vi "VisualCheckSubPanel.vi"(6 "GuiRef":T1={"StringOut"=refnum, "AbortOnFail"=refnum, "SN"=refnum, "SN_Length"=refnum, "TestResult"=refnum, "CycleTime"=refnum, "ErrorCode"=refnum, "UUTStatus"=refnum, "DataBaseEnable?"=refnum, "DUTModel"=refnum, "FixtureID"=refnum, "OperatorID"=refnum, "SNReady"=refnum, "StopSlot"=refnum, "NextStep"=refnum, "PassYeild"=refnum, "Failed"=refnum, "Passed"=refnum, "Tested"=refnum, "TestItemsCtl"={"StepName"="", "TestEnable"=FALSE, "LoopCount"=0, "StopOnFail"=FALSE, "Index"=0, "TestName"="", "通道"="", "参数"="", "TimeStart"=0}, "ProcessBar"=refnum, "Slot"=enum."Slot1", "Row"=3, "States"=refnum, "TestMode"=refnum, "循环次数-DUT"=refnum, "波形图"=refnum, "产品型号"=refnum, "子面板"=refnum, "测试失败项目"=refnum, "测试结果"=refnum, "DUT"=refnum, "Starttime"=refnum, "SlotReady"=refnum, "版本信息"=refnum, "WIFI_1"=refnum, "WIFI_2"=refnum, "直通率"=refnum, "卡1开卡结果"=refnum, "卡2开卡结果"=refnum}, 8 "error in (no error)":errorcluster, 10 "测试项":string) -> (0 "error out":errorcluster, 2 "StringOut":string, 3 "Result":bool)   [LabVIEW 2013]
uses:
  SystemCode/SysControl/Reference.ctl
  SystemCode/SysControl/TestItemsCTL.ctl
  SystemCode/SysControl/Slot.ctl
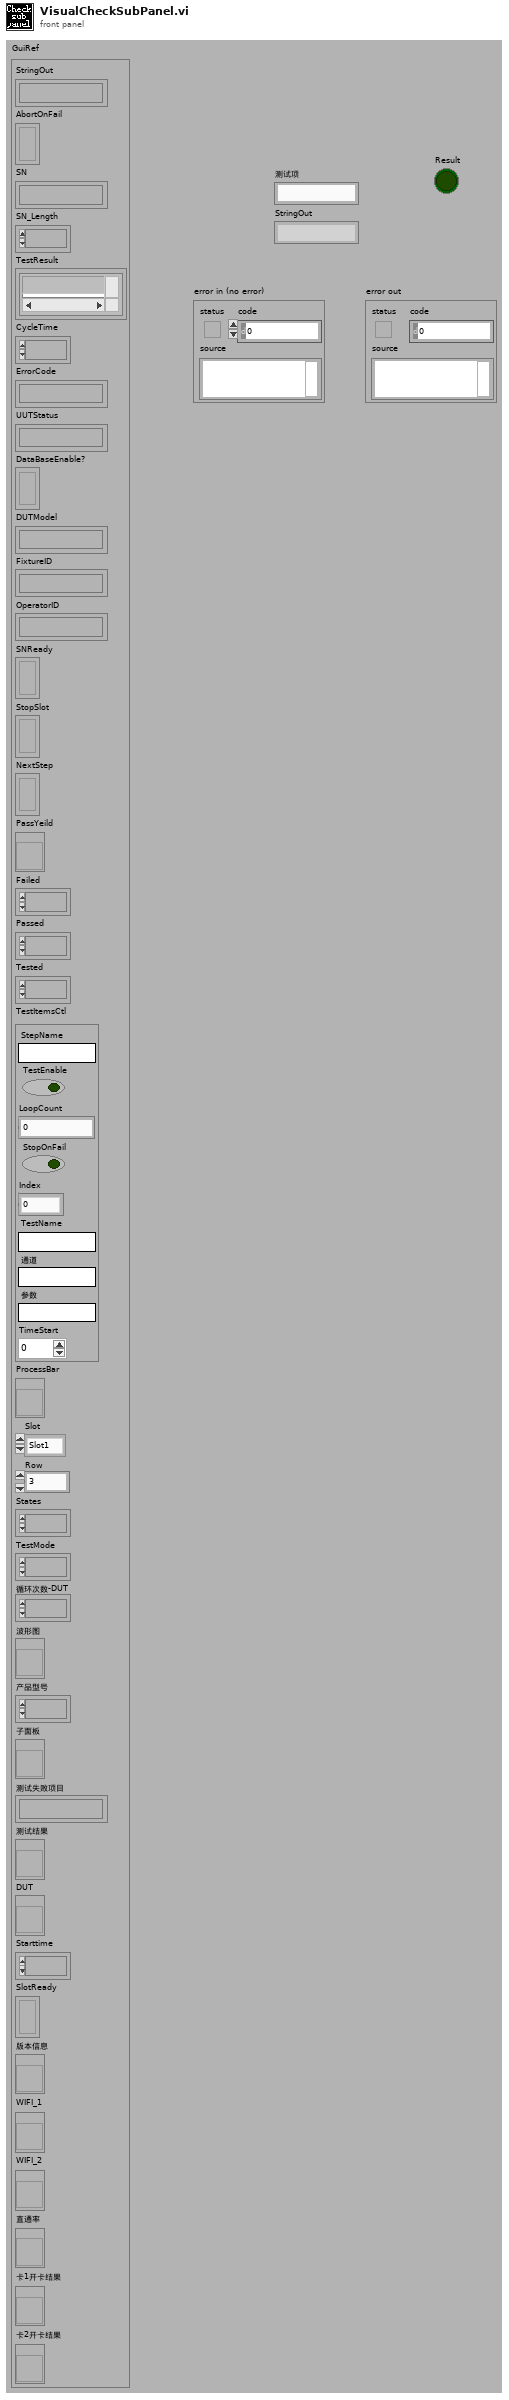
[diagram p1: front panel]
types:
  T1 = typedef "Reference.ctl" = cluster{"StringOut":refnum<vi>, "AbortOnFail":refnum<vi>, "SN":refnum<vi>, "SN_Length":refnum<vi>, "TestResult":refnum<vi>, "CycleTime":refnum<vi>, "ErrorCode":refnum<vi>, "UUTStatus":refnum<vi>, "DataBaseEnable?":refnum<vi>, "DUTModel":refnum<vi>, "FixtureID":refnum<vi>, "OperatorID":refnum<vi>, "SNReady":refnum<vi>, "StopSlot":refnum<vi>, "NextStep":refnum<vi>, "PassYeild":refnum<vi>, "Failed":refnum<vi>, "Passed":refnum<vi>, "Tested":refnum<vi>, "TestItemsCtl":T2, "ProcessBar":refnum<vi>, "Slot":T3, "Row":u32, "States":refnum<vi>, "TestMode":refnum<vi>, "循环次数-DUT":refnum<vi>, "波形图":refnum<vi>, "产品型号":refnum<vi>, "子面板":refnum<vi>, "测试失败项目":refnum<vi>, "测试结果":refnum<vi>, "DUT":refnum<vi>, "Starttime":refnum<vi>, "SlotReady":refnum<vi>, "版本信息":refnum<vi>, "WIFI_1":refnum<vi>, "WIFI_2":refnum<vi>, "直通率":refnum<vi>, "卡1开卡结果":refnum<vi>, "卡2开卡结果":refnum<vi>}
  T2 = typedef "TestItemsCTL.ctl" = cluster{"StepName":string, "TestEnable":bool, "LoopCount":i32, "StopOnFail":bool, "Index":u32, "TestName":string, "通道":string, "参数":string, "TimeStart":u32}
  T3 = typedef "Slot.ctl" = enum16{"Slot1", "Slot2", "Slot3", "Slot4"}
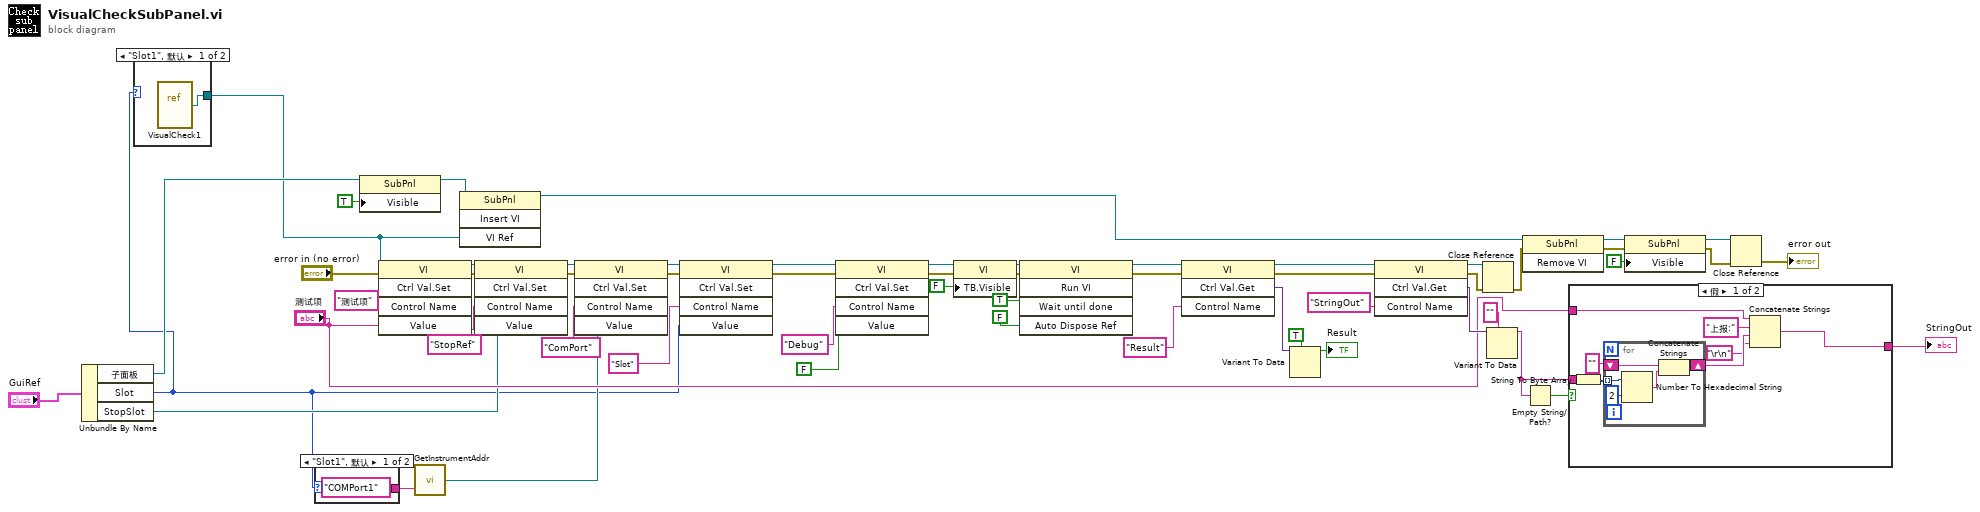
[diagram p0: block diagram]
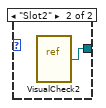
[diagram p2: hidden frame]
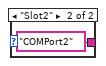
[diagram p3: hidden frame]
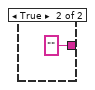
[diagram p4: hidden frame]
diagram:
  n1 = Unbundle By Name("GuiRef") -> ("子面板"=w17:refnum<vi>, "Slot"=w3:T3, "StopSlot"=w4:refnum<vi>)
  n2 = case shown="\"Slot1\", 默认" w3 {
    tunnel: [w57 w58] -> w10
    frame "Slot1", Default {
      n3 = vi-ref "VisualCheck1.vi"() -> (w57:refnum<vi>)
    }
    frame "Slot2" {
      n4 = vi-ref "VisualCheck2.vi"() -> (w58:refnum<vi>)
    }
  }
  n5 = case shown="\"Slot1\", 默认" w3 {
    tunnel: ["COMPort1" ("String") "COMPort2" ("String")] -> w16
    frame "Slot1", Default {
    }
    frame "Slot2" {
    }
  }
  n6 = property class="SubPnl"(reference=w17, "Visible"=TRUE ("可见")) -> (reference out=w44:refnum<vi>)  [unwired: 1 in, 1 out]
  n7 = invoke class="VI" method="Ctrl Val.Set"(reference=w10, error in="error in (no error)", "Control Name"="测试项", "Value"="测试项") -> (reference out=w7:refnum<vi>, error out=w8:errorcluster)  [unwired: 1 in, 3 out]
  n8 = call "GetInstrumentAddr.vi"("String"=w16) -> ("VISA session"=w15:refnum<visa-resource-name>)  [unwired: 1 out]
  n9 = invoke on="Invoke Node" class="SubPnl" method="Insert VI"(reference=w44, "VI Ref"=w10) -> (reference out=w43:refnum<vi>)  [unwired: 2 in, 3 out]
  n10 = invoke class="VI" method="Ctrl Val.Set"(reference=w7, error in=w8, "Control Name"="StopRef" ("控件名"), "Value"=w4) -> (reference out=w6:refnum<vi>, error out=w5:errorcluster)  [unwired: 1 in, 3 out]
  n11 = invoke class="VI" method="Ctrl Val.Set"(reference=w6, error in=w5, "Control Name"="ComPort" ("控件名"), "Value"=w15) -> (reference out=w22:refnum<vi>, error out=w19:errorcluster)  [unwired: 1 in, 3 out]
  n12 = invoke class="VI" method="Ctrl Val.Set"(reference=w22, error in=w19, "Control Name"="Slot" ("控件名"), "Value"=w3) -> (reference out=w2:refnum<vi>, error out=w1:errorcluster)  [unwired: 1 in, 3 out]
  n13 = invoke class="VI" method="Ctrl Val.Set"(reference=w2, error in=w1, "Control Name"="Debug" ("控件名"), "Value"=FALSE ("前面板窗口:显示菜单栏")) -> (reference out=w13:refnum<vi>, error out=w14:errorcluster)  [unwired: 1 in, 3 out]
  n14 = property class="VI"(reference=w13, error in=w14, "TB.Visible"=FALSE ("前面板窗口:显示菜单栏")) -> (reference out=w35:refnum<vi>, error out=w34:errorcluster)
  n15 = invoke class="VI" method="Run VI"(reference=w35, error in=w34, "Wait until done"=TRUE ("Wait Until Done"), "Auto Dispose Ref"=FALSE ("Auto Dispose Reference")) -> (reference out=w48:refnum<vi>, error out=w47:errorcluster)  [unwired: 1 in, 3 out]
  n16 = invoke class="VI" method="Ctrl Val.Get"(reference=w48, error in=w47, "Control Name"="Result") -> (reference out=w32:refnum<vi>, error out=w31:errorcluster, "Get Control Value Variant"=w56:variant)  [unwired: 1 in, 1 out]
  n17 = Variant To Data(type=TRUE ("Key1"), Variant=w56) -> (data=→"Result":bool)  [unwired: 1 in, 1 out]
  n18 = invoke class="VI" method="Ctrl Val.Get"(reference=w32, error in=w31, "Control Name"="StringOut") -> (reference out=w30:refnum<vi>, error out=w29:errorcluster, "Get Control Value Variant"=w28:variant)  [unwired: 1 in, 1 out]
  n19 = Close Reference(reference=w30, error in (no error)=w29) -> (error out=w50:errorcluster)
  n20 = Variant To Data(type="" ("Control Name"), Variant=w28) -> (data=w26:string)  [unwired: 1 in, 1 out]
  n21 = invoke on="Invoke Node" class="SubPnl" method="Remove VI"(reference=w43, error in=w50) -> (reference out=w39:refnum<vi>, error out=w40:errorcluster)  [unwired: 1 in, 1 out]
  n22 = Empty String/Path?(string/path=w26) -> (empty?=w25:bool)
  n23 = case shown="假" w25 {
    tunnel: w26 -> [w63 _]
    tunnel: [w62 ""] -> w24
    tunnel: "测试项" -> [w61 _]
    frame False {
      n24 = String To Byte Array(string=w63) -> (unsigned byte array=w68:u8[])
      n25 = for "For循环" {
        tunnel: w68 -> [w73] mode=indexing
        shift-right: [w71] -> w65
        shift-left: "" -> [w70]
        n26 = Number To Hexadecimal String(1:i16 2 ("宽度(-)"), 2:w73) -> (0:w72:string)
        n27 = Concatenate Strings(w70, w72) -> (w71:string)
      }
      n28 = Concatenate Strings(w61, "上报:" ("字符串"), w65, "\r\n") -> (w62:string)
    }
    frame True {
    }
  }
  "StringOut" <- w24
  n29 = property class="SubPnl"(reference=w39, error in=w40, "Visible"=FALSE ("可见")) -> (reference out=w37:refnum<vi>, error out=w38:errorcluster)
  n30 = Close Reference(reference=w37, error in (no error)=w38) -> (error out=→"error out":errorcluster)
